vi "Get Matrix String.vi"(10 "matrix key":string, 11 "info data":string) -> (1 "key found?":bool, 3 "matrix part":string)   [LabVIEW 2020, in "infolib.lvlib"]
doc: "Finds matrix denoted by <b>matrix key</b> in string <b>info data</b> and returns the value of the matrix. If the key is found, the <b>key found?</b> output is true even if the matrix itself is empty."
uses:
  infolib.lvlib
  <vilib>/regexp/Match Regular Expression.xnode
panel:
  out "regexp":string
  # "testing string:"
  # "blfdablad\n#startmatrix:: a\n1; 2; 3;\n#endmatrix:: a\n#startsection:: 1\n   #startmatrix:: b\n   1; 2; 3;\n  4;   5 ; 6   ;\n   #endmatrix:: b\n#endsection:: 1\njfdklajfkdl"
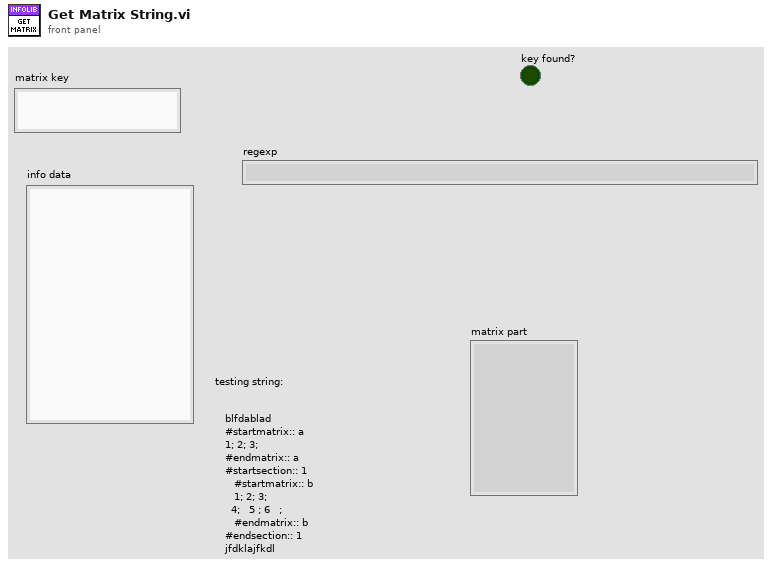
[diagram p1: front panel]
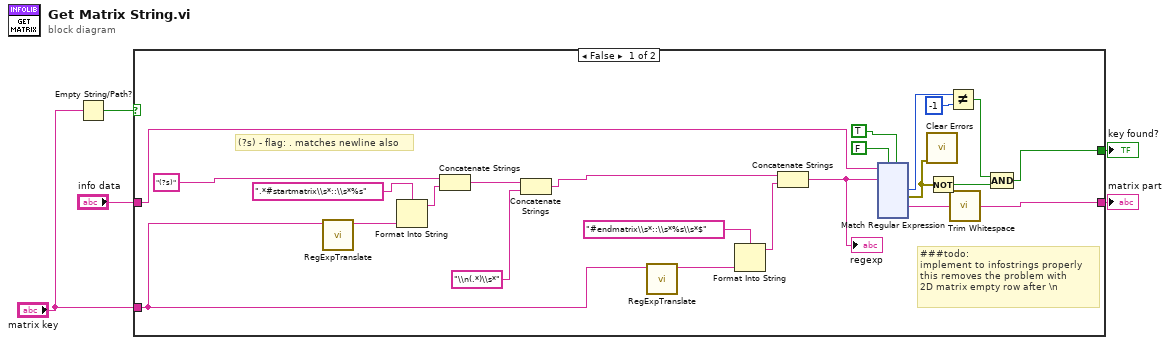
[diagram p0: block diagram]
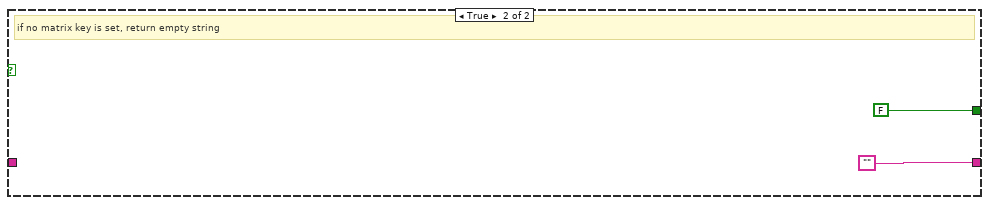
[diagram p2: hidden frame]
diagram:
  n1 = Empty String/Path?(string/path="matrix key") -> (empty?=w3:bool)
  n2 = case shown="False" w3 {
    tunnel: [w20 FALSE] -> w5
    tunnel: [w6 ""] -> w4
    tunnel: "info data" -> [w14 _]
    tunnel: "matrix key" -> [w13 _]
    frame False {
      # "###todo:\nimplement to infostrings properly\nthis removes the problem with \n2D matrix empty row after \\n"
      # "(?s) - flag: . matches newline also"
      n3 = call "RegExpTranslate.vi"("string"=w13) -> ("regexp safe string"=w10:string)  [unwired: 10 in]
      n4 = Format Into String(format string=".*#startmatrix\\s*::\\s*%s", w10) -> (resulting string=w11:string)  [unwired: 2 in, 1 out]
      n5 = Concatenate Strings("(?s)" ("section name"), w11) -> (w23:string)
      n6 = Concatenate Strings(w23, "\\n(.*)\\s*" ("string")) -> (w21:string)
      n7 = call "RegExpTranslate.vi"("string"=w13) -> ("regexp safe string"=w7:string)  [unwired: 10 in]
      n8 = Format Into String(format string="#endmatrix\\s*::\\s*%s\\s*$", w7) -> (resulting string=w8:string)  [unwired: 2 in, 1 out]
      n9 = Concatenate Strings(w21, w8) -> (w16:string)
      "regexp" <- w16
      n10 = xnode "Match Regular Expression"("input string"=w14, "regular expression"=w16, "ignore case? (F)"=FALSE, "multiline? (F)"=TRUE) -> ("offset past match"=w25:i32, "error out"=w17:errorcluster, "submatch 1"=w15:string)  [unwired: 2 in, 4 out]
      n11 = call <vilib>:"Clear Errors.vi"("error in (no error)"=w17) -> ()  [unwired: 5 in, 2 out]
      n12 = Not(x=w17) -> (.not. x?=w18:bool)
      n13 = Not Equal?(x=w25, y=-1 ("x")) -> (x != y?=w19:bool)
      n14 = call <vilib>:"Trim Whitespace.vi"("string"=w15) -> ("trimmed string"=w6:string)  [unwired: 1 in]
      n15 = Compound Arithmetic op=AND(w19, w18) -> (w20:bool)
    }
    frame True {
      # "if no matrix key is set, return empty string"
    }
  }
  "key found?" <- w5
  "matrix part" <- w4
